vi "faux_daq.vi"() -> ()   [LabVIEW 2022 SP3]
panel:
  in  "Select Module":enum16{"motion", "Motor Class"}(ring)
  out "Outputs":T1(array[cluster])
  in  "Requests":cluster{"Request":string, "Payload":string}[](array[cluster])=[{"Request"="initialize", "Payload"="192.168.6.104"}, {"Request"="move_to", "Payload"="200000"}, {"Request"="move_to", "Payload"="100000"}, {"Request"="move_to", "Payload"="0"}, {"Request"="move_to", "Payload"="-100000"}, {"Request"="move_to", "Payload"="-200000"}, {"Request"="cleanup", "Payload"=""}]
  out "error out":errorcluster
  in  "error in":errorcluster
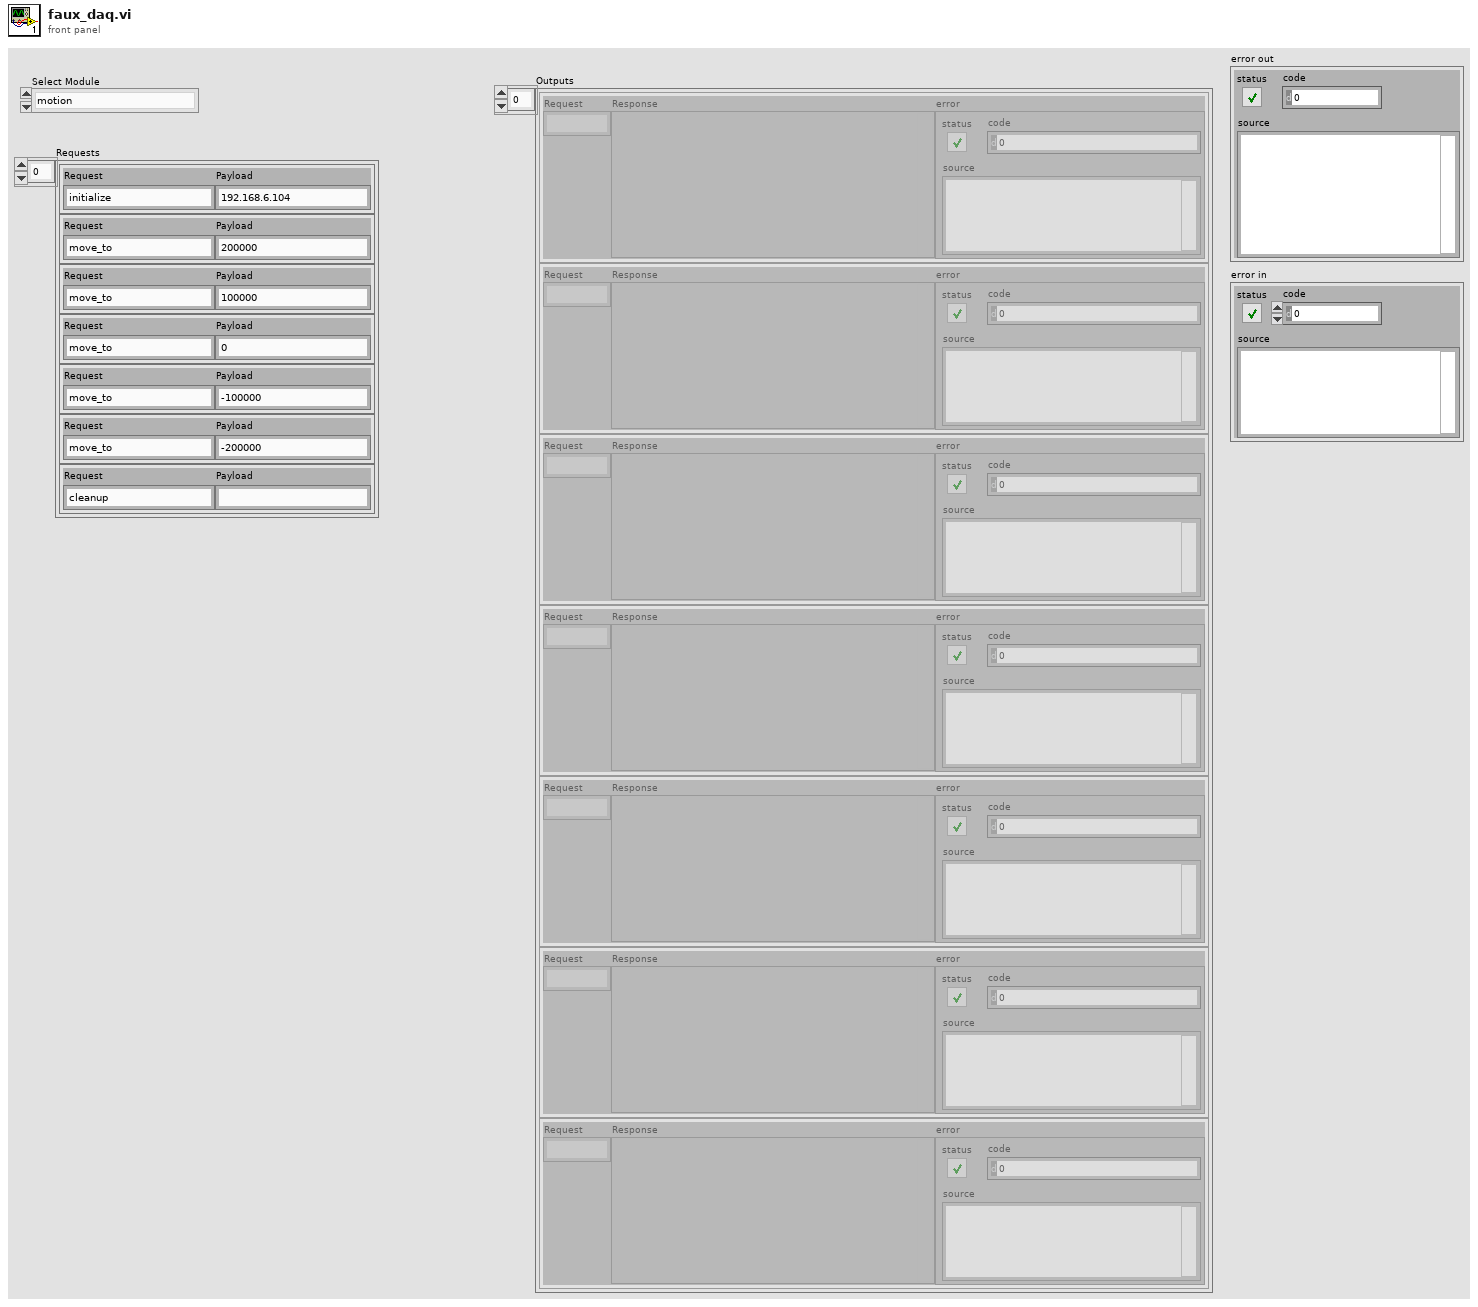
[diagram p1: front panel]
types:
  T1 = cluster{"Request":string, "Response":variant, "error":errorcluster}[]
  T2 = cluster{"Request":string, "Response":variant, "error":errorcluster}
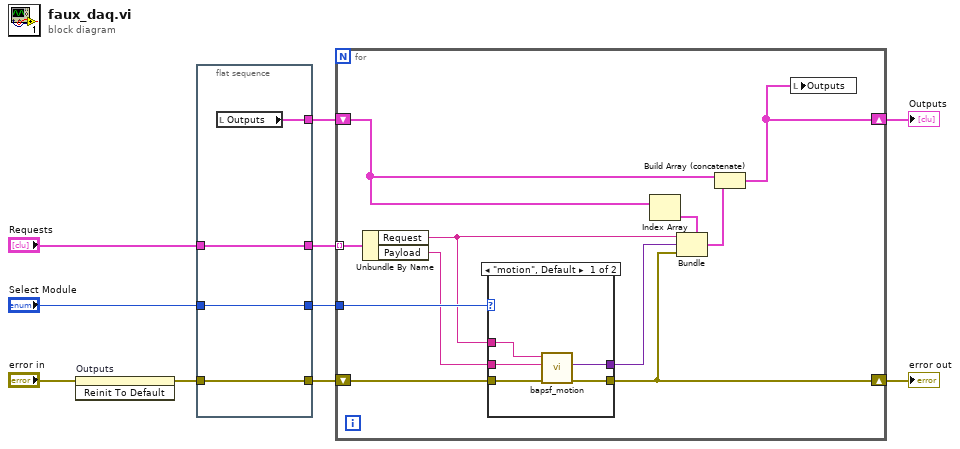
[diagram p0: block diagram]
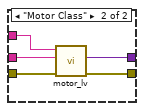
[diagram p2: hidden frame]
diagram:
  n1 = invoke on="Outputs" class="Arr (strict)" method="Reinit To Default"(error in="error in") -> (error out=w6:errorcluster)  [unwired: 2 in, 2 out]
  n2 = flat-sequence {
    tunnel: [w14] -> w7
    tunnel: w6 -> [w14]
    tunnel: [w13] -> w5
    tunnel: "Requests" -> [w12]
    tunnel: [w12] -> w3
    tunnel: "Select Module" -> [w11]
    tunnel: [w11] -> w1
    frame #0 {
      n3 = local read "Outputs"() -> (w13:T1)
    }
  }
  n4 = for {
    tunnel: w3 -> [w18] mode=indexing
    shift-right: [w20] -> w10
    shift-left: w7 -> [w25]
    shift-right: [w15] -> w9
    shift-left: w5 -> [w23]
    tunnel: w1 -> [w19]
    n5 = Unbundle By Name(w18) -> ("Request"=w16:string, "Payload"=w17:string)
    n6 = case shown="\"motion\", Default" w19 {
      tunnel: w25 -> [w30 w35]
      tunnel: [w29 w33] -> w21
      tunnel: [w28 w34] -> w20
      tunnel: w17 -> [w27 w32]
      tunnel: w16 -> [w26 w31]
      frame "motion", Default {
        n7 = call "bapsf_motion.vi"("error in"=w30, "Request data"=w27, "Request"=w26) -> ("error out"=w28:errorcluster, "Response data"=w29:variant)  [unwired: 3 in]
      }
      frame "Motor Class" {
        n8 = call "motor_lv.vi"("error in"=w35, "Request data"=w32, "Request"=w31) -> ("error out"=w34:errorcluster, "Response data"=w33:variant)  [unwired: 3 in]
      }
    }
    n9 = Index Array(array=w23) -> (element=w22:T2)  [unwired: 1 in]
    n10 = Bundle(cluster=w22, "Request"=w16, "Response"=w21, "error"=w20) -> (w24:T2)
    n11 = Build Array (concatenate)(w23, w24) -> (w15:T1)
    n12 = local write "Outputs"(w15) -> ()
  }
  "error out" <- w10
  "Outputs" <- w9
